vi "Pressure_Test_V1.vi"() -> ()   [LabVIEW 2015]
uses:
  <vilib>/express/express analysis/Spectral/Block/exnSpectralBlock spectral measurements power poly.vi
  <vilib>/express/express analysis/Spectral/Block/exnSpectralBlock spectral measurements power DDT.vi
  <vilib>/express/express analysis/Spectral/XNode/ExpressSpectralMeasurementsBlockNode.xnode
  <vilib>/Analysis/NI_AALBase.lvlib
panel:
  in  "cycles 3":dbl=1.0 format="%0.2f"
  in  "cycles 2":dbl=1.0 format="%0.2f"
  in  "cycles":dbl=1.0 format="%0.2f"
  in  "amplitude":dbl=1.0 format="%0.2f"
  in  "samples 3":i32=128
  in  "amplitude 2":dbl=1.0 format="%0.2f"
  in  "samples 2":i32=128
  out "Waveform Graph":dynamicdata(graph)
  in  "phase in":dbl format="%0.2f"
  in  "frequency":dbl=0.0078125 format="%0.4e"
  in  "stop":bool
  in  "Boolean":bool
  in  "Path":path
  out "Waveform Chart":dynamicdata(graph)
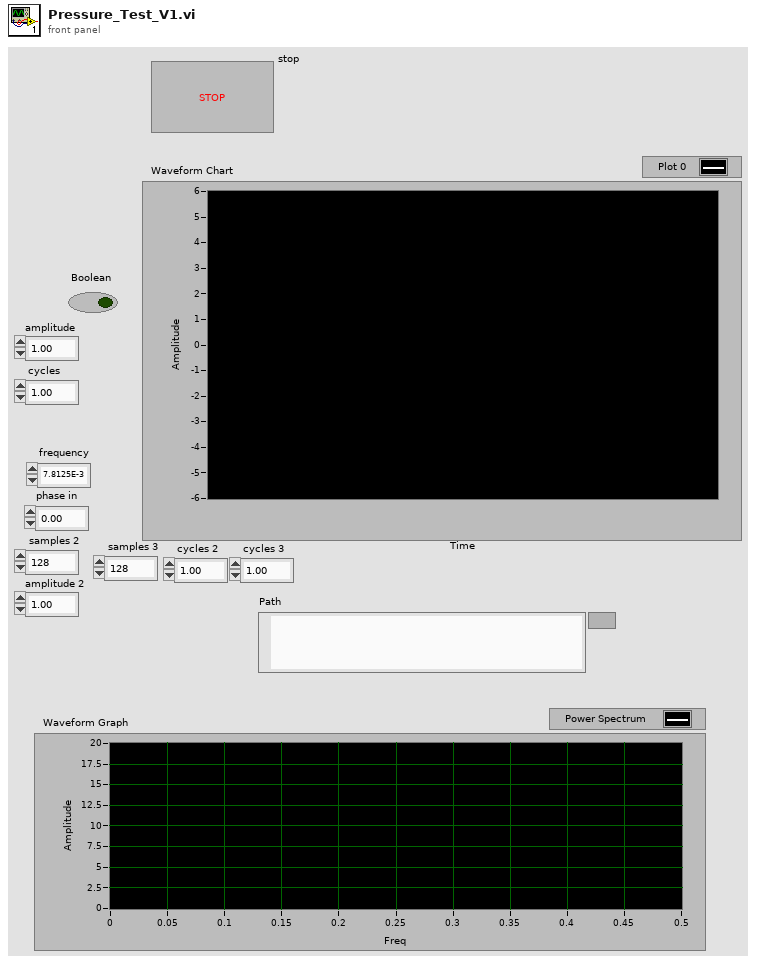
[diagram p1: front panel]
types:
  T1 = cluster{"averaging mode":u16, "weighting mode":u16, "number of averages":u32}
  T2 = cluster{"dB On (F)":bool, "unwrap phase (F)":bool, "convert to degree (F)":bool}
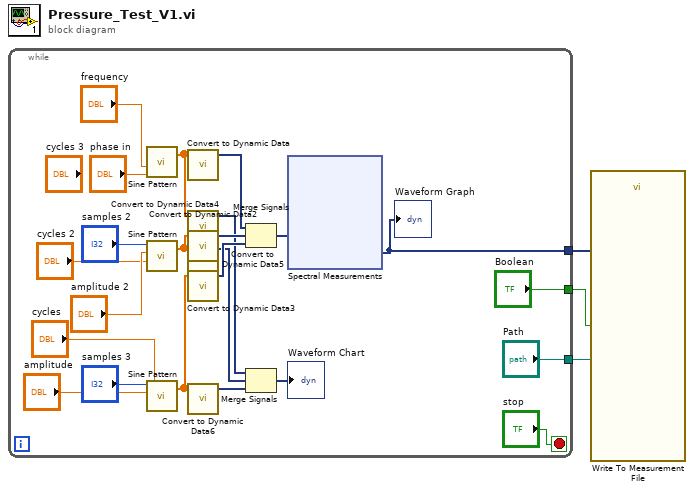
[diagram p0: block diagram]
diagram:
  n1 = while {
    tunnel: ["Boolean"] -> w3
    tunnel: ["Path"] -> w2
    tunnel: [w4] -> w1
    stop <- "stop" stop-if-true
    n2 = call <vilib>:"Sine Pattern.vi"("cycles"="phase in", "phase(degrees)"="frequency") -> ("Sinusoidal Pattern"=w14:dbl[])  [unwired: 2 in, 1 out]
    n3 = call <vilib>:"Sine Pattern.vi"("cycles"="cycles 2", "amplitude"="amplitude 2", "samples"="samples 2") -> ("Sinusoidal Pattern"=w11:dbl[])  [unwired: 1 in, 1 out]
    n4 = call <vilib>:"Sine Pattern.vi"("cycles"="cycles", "amplitude"="amplitude", "samples"="samples 3") -> ("Sinusoidal Pattern"=w9:dbl[])  [unwired: 1 in, 1 out]
    n5 = call "Convert to Dynamic Data"("Array"=w14) -> ("Dynamic Data Type"=w20:dynamicdata)  [unwired: 3 in]
    n6 = call "Convert to Dynamic Data4"("Array"=w14) -> ("Dynamic Data Type"=w13:dynamicdata)  [unwired: 3 in]
    n7 = call "Convert to Dynamic Data2"("Array"=w11) -> ("Dynamic Data Type"=w19:dynamicdata)  [unwired: 3 in]
    n8 = call "Convert to Dynamic Data5"("Array"=w11) -> ("Dynamic Data Type"=w10:dynamicdata)  [unwired: 3 in]
    n9 = call "Convert to Dynamic Data3"("Array"=w9) -> ("Dynamic Data Type"=w18:dynamicdata)  [unwired: 3 in]
    n10 = call "Convert to Dynamic Data6"("Array"=w9) -> ("Dynamic Data Type"=w8:dynamicdata)  [unwired: 3 in]
    n11 = Merge Signals(w20, w19, w18) -> (w21:dynamicdata)
    n12 = Merge Signals(w13, w10, w8) -> (→"Waveform Chart":dynamicdata)
    n13 = xnode "Spectral Measurements"("Signals"=w21) -> ("Power Spectrum"=w4:dynamicdata)  [unwired: 1 in, 1 out]
    "Waveform Graph" <- w4
  }
  n14 = call "Write To Measurement File"("Signals"=w1, "Enable"=w3, "Filename"=w2) -> ()  [unwired: 14 in, 3 out]
